vi "Control Drive.vi"(9 "X-DriveAuto":dbl, 11 "Y-DriveAuto":dbl) -> ()   [LabVIEW 2020]
uses:
  Framework/Robot Global Data.vi
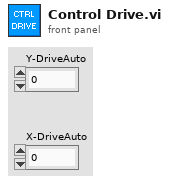
[diagram p1: front panel]
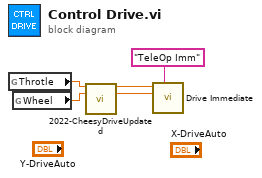
[diagram p0: block diagram]
diagram:
  n1 = global read "Robot Global Data.vi" "Throtle"() -> (w4:dbl)
  n2 = global read "Robot Global Data.vi" "Wheel"() -> (w5:dbl)
  n3 = call "2022-CheesyDriveUpdated.vi"("Throttle"=w4, "Wheel"=w5) -> ("Left PWM"=w2:dbl, "Right PWM"=w3:dbl)  [unwired: 11 in, 1 out]
  n4 = call "Drive Immediate.vi"("Description"="TeleOp Imm", "Right Setpoint"=w3, "Left Setpoint"=w2) -> ()  [unwired: 8 in, 1 out]
